vi "AVTCP-Clear FGVs.vi"   [LabVIEW 2020]
uses:
  AVTCP-FGV Action.ctl
types:
  T1 = typedef "AVTCP-FGV Action.ctl" = enum16{"Init", "Write", "Read"}
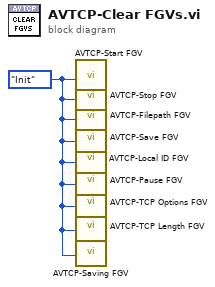
[diagram p0: block diagram]
diagram:
  w1 = AVTCP-FGV_Action."Init" ("Action")
  n1 = call "AVTCP-Start FGV.vi"("Action"=w1) -> ()  [unwired: 6 in, 1 out]
  n2 = call "AVTCP-Stop FGV.vi"("Action"=w1) -> ()  [unwired: 6 in, 1 out]
  n3 = call "AVTCP-Filepath FGV.vi"("Action"=w1) -> ()  [unwired: 6 in, 1 out]
  n4 = call "AVTCP-Save FGV.vi"("Action"=w1) -> ()  [unwired: 6 in, 1 out]
  n5 = call "AVTCP-Local ID FGV.vi"("Action"=w1) -> ()  [unwired: 5 in, 2 out]
  n6 = call "AVTCP-Pause FGV.vi"("Action"=w1) -> ()  [unwired: 6 in, 1 out]
  n7 = call "AVTCP-TCP Options FGV.vi"("Action"=w1) -> ()  [unwired: 5 in, 2 out]
  n8 = call "AVTCP-TCP Length FGV.vi"("Action"=w1) -> ()  [unwired: 6 in, 1 out]
  n9 = call "AVTCP-Saving FGV.vi"("Action"=w1) -> ()  [unwired: 6 in, 1 out]
